vi "dfd_Lattice Allpass Normalization (OneM).vi"(7 "scale type":T1, 10 "coefficients k":dbl[](array[numeric]) format="%.2f", 11 "x":dbl[](array[numeric])) -> (2 "norm":dbl[](array[numeric]) format="%.2f", 3 "y":dbl[](array[numeric]))   [LabVIEW 2017, in "NI_DigFilter_FXP.lvlib"]
uses:
  <vilib>/addons/Digital Filter Design/NI_DigFilter_FXP.lvlib
  <vilib>/addons/Digital Filter Design/_Objects.llb/DFD Coef Norm Type.ctl
  <vilib>/addons/Digital Filter Design/NI_DigFilterLicensed.lvlib
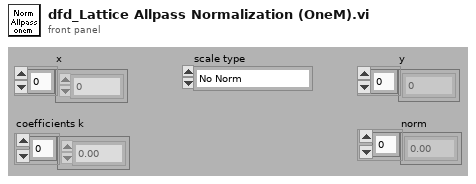
[diagram p1: front panel]
types:
  T1 = typedef "NI_DigFilterLicensed.lvlib/DFD Coef Norm Type.ctl" = enum16{"No Norm", "Time Domain 1-Norm", "Time Domain 2-Norm", "Time Domain Inf-Norm"}
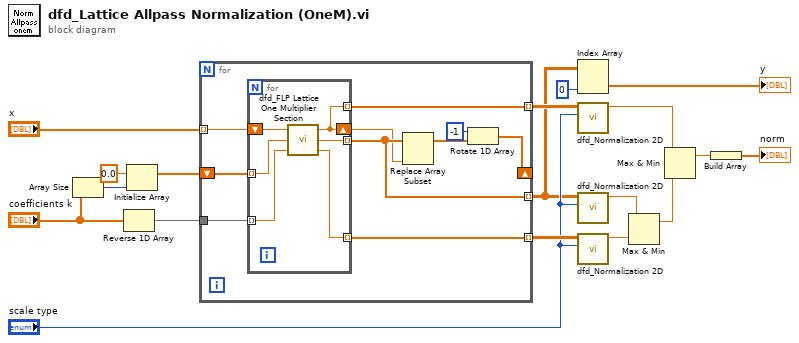
[diagram p0: block diagram]
diagram:
  n1 = Array Size(array="coefficients k") -> (size(s)=w16:i32)
  n2 = Reverse 1D Array(array="coefficients k") -> (reversed array=w15:dbl[])
  n3 = Initialize Array(0.0 ("element"), w16) -> (w18:dbl[])
  n4 = for {
    tunnel: w15 -> [w28]
    shift-right: [w27] -> _
    shift-left: w18 -> [w26]
    tunnel: [w23] -> w3 mode=indexing
    tunnel: [w25] -> w11 mode=indexing
    tunnel: [w24] -> w10 mode=indexing
    tunnel: "x" -> [w22] mode=indexing
    n5 = for {
      shift-right: [w30] -> w21
      shift-left: w22 -> [w34]
      tunnel: w26 -> [w33] mode=indexing
      tunnel: w28 -> [w32] mode=indexing
      tunnel: [w31] -> w23 mode=indexing
      tunnel: [w30] -> w25 mode=indexing
      tunnel: [w29] -> w24 mode=indexing
      n6 = call <vilib>:"dfd_FLP Lattice One Multiplier Section.vi"("k(m)"=w32, "w(m-1)"=w33, "x(m)"=w34) -> ("u(m)"=w29:dbl, "w(m)"=w31:dbl, "x(m-1)"=w30:dbl)
    }
    n7 = Replace Array Subset(array=w23, new element=w21) -> (w20:dbl[])  [unwired: 1 in]
    n8 = Rotate 1D Array(1:w20, 2:-1 ("n")) -> (0:w27:dbl[])
  }
  n9 = Index Array(array=w3, index (col)=0 ("disabled index (col)")) -> (element=→"y":dbl[])  [unwired: 1 in]
  n10 = call <vilib>:"dfd_Normalization 2D.vi"("scale type"="scale type", "2D Array (col-major)"=w11) -> ("max norm"=w5:dbl)  [unwired: 9 out]
  n11 = call <vilib>:"dfd_Normalization 2D.vi"("scale type"="scale type", "2D Array (col-major)"=w3) -> ("max norm"=w8:dbl)  [unwired: 9 out]
  n12 = call <vilib>:"dfd_Normalization 2D.vi"("scale type"="scale type", "2D Array (col-major)"=w10) -> ("max norm"=w7:dbl)  [unwired: 9 out]
  n13 = Max & Min(x=w8, y=w7) -> (max(x,y)=w6:dbl)  [unwired: 1 out]
  n14 = Max & Min(x=w5, y=w6) -> (max(x,y)=w4:dbl)  [unwired: 1 out]
  n15 = Build Array(w4) -> (→"norm":dbl[])
